vi "SCMP - System init v2.vi"(8 "error in (no error)":errorcluster, 9 "Pane Color":u32, 10 "instrument":string) -> (0 "error main":errorcluster, 1 "Cameras":refnum<class "Camera.lvclass">[](array[class]), 2 "Peripherals":T1, 3 "cont?":bool=TRUE, 5 "Today's SCMP Engineering File":path, 7 "Version":string)   [LabVIEW 2014]
uses:
  Controls/peripherals.ctl
  AISAS/Mech/AISAS Mech.lvclass
  Camera/Camera/Camera.lvclass
  Camera/Andor Neo/Andor.lvclass
  Controls/SCD - FITS Cluster.ctl
  AISAS/Controls/Diffuser.ctl
  Controls/FITS Data type.ctl
  Controls/SCD - Calibration Optics Filter Wheel.ctl
  Controls/SCD - EDT - Emission Line Filter Wheel.ctl
  Controls/CoMP-S Controls/Polarization Optics Filter Wheel.ctl
  Controls/CoMP-S Controls/Emission Line Filter Wheel.ctl
  AISAS/Controls/focus.ctl
  Controls/Cameras select.ctl
  Controls/Globals.vi
  Controls/Global demo.vi
panel:
  in  "Force PI Init":bool
  in  "Shutter":string(combo)="Global"
  in  "Temperature":string(combo)="-25.00"
  out "error eng":errorcluster
  # "System initialization\n        wait please"
  # "Peripherals"
  # "Andor control"
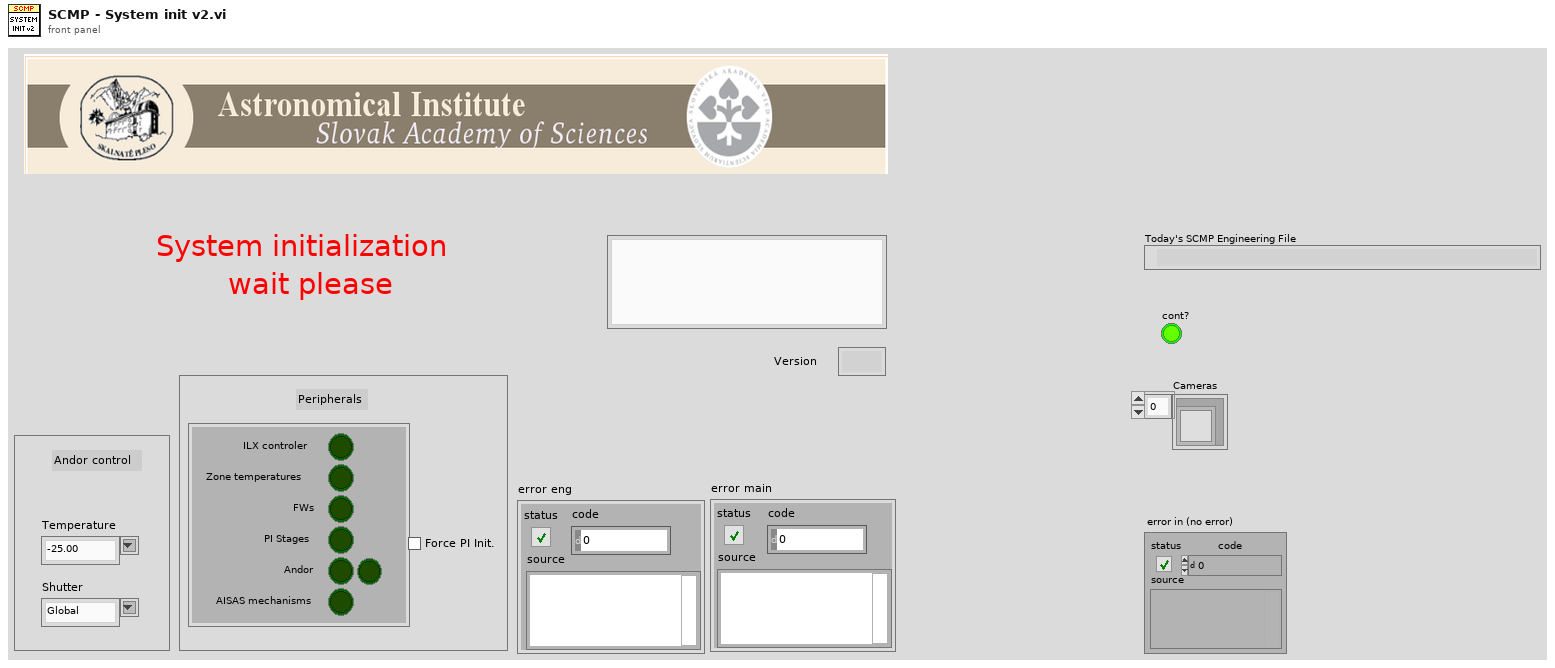
[diagram p1: front panel]
types:
  T1 = typedef "peripherals.ctl" = cluster{"ILX controler":bool, "Zone temperatures":bool, "Andor":bool, "Andor 2":bool, "PI Stages":bool, "AISAS mechanisms":bool, "AISAS Mech.lvclass":refnum<class "AISAS Mech.lvclass">, "Zone temp ref":variant, "FWs":bool}
  T2 = cluster{"server address":string, "remote port (502)":u16}
  T3 = enum32{"Invalid", "Standard", "Closed", "Hidden", "Minimized", "Maximized"}
  T4 = typedef "SCD - FITS Cluster.ctl" = cluster{"Wavelength (nm)":dbl, "Exposure (s)":dbl, "Tuning Delay (ms)":dbl, "Beam Type (-1/1)":dbl, "Tuning Voltages":dbl[], "Observer":string, "Light Shapping Diffuser":T5, "Comment":string, "Data Type":T6, "Mod Cycles":u16, "SCD Calibration Optics":T7, "SCD Emission Line Filter":T8, "Cookbook":string, "COMP-S Calibration Wheel":T9, "COMP-S Andover Filter Wheel":T10, "FOV Rotation (deg)":dbl, "Objective Lens Position (mm)":T11, "Occulter size":dbl, "Time End":timestamp, "Acc Exposure (s)":dbl, "Time Stamp Array":timestamp[], "Camera Serial Number":string[], "Camera Temp":dbl[], "Camera PI (mm)":dbl[], "Time Start":timestamp, "Peripherals":T1, "FITS paths":path[], "Cameras":T12, "load preset cbk":bool, "periodic check count":i32, "COMP-S Calibration Wheel 2":T9, "Calib":enum16{"Dark", "Flat"}, "Abso Aperture":dbl, "Nominal Aperture":dbl, "Pointer IP":string}
  T5 = typedef "Diffuser.ctl" = enum16{"Out of Beam", "In Beam"}
  T6 = typedef "FITS Data type.ctl" = enum16{"LIVE", "DARK", "FLAT", "CALI", "OBSE", "ABSO", "AURE", "TARG", "OBJE", "HOLE", "OREX", "THRO", "CHIP"}
  T7 = typedef "SCD - Calibration Optics Filter Wheel.ctl" = enum16{"1 - Polarizer @0, I+Q", "2 - Polarizer @90, I-Q", "3 - Polarizer @45, I+U", "4 - Polarizer @135, I-U", "5 - Polarizer @0, Retarder @45, I+V", "6 - Polarizer @0, Retarder @135, I-V", "7 - Dark", "8 - Clear", "9 - N/A"}
  T8 = typedef "SCD - EDT - Emission Line Filter Wheel.ctl" = enum16{"1-557.6nm", "2-587.6nm", "3-589.6nm", "4-630.2nm", "5-656.4nm", "6-849.8nm", "7-854.2nm", "8-866.2nm", "9-1083.0nm"}
  T9 = typedef "Polarization Optics Filter Wheel.ctl" = enum16{"Dark", "Clear", "Exchange Lens", "Polarizer @0, I+Q", "Polarizer @90, I-Q", "Polarizer @45, I+U", "Polarizer @135, I-U", "Polarizer @0, Retarder @45, I+V", "Polarizer @0, Retarder @135, I-V"}
  T10 = typedef "Emission Line Filter Wheel.ctl" = enum16{"530.3nm/HWB 0.34nm (Fe XIV)", "587.6nm/HBW 0.44nm (He I D3)", "637.5nm/HBW 0.53nm (Fe X)", "656.3nm/HBW 0.57nm (H-Alpha)", "789.2nm/HBW 0.85nm (Fe XI)", "854.2nm/HBW 1.01nm (Ca I)", "1074.7nm/HBW 2.34nm (Fe XIII)", "1079.8nm/HBW 1.64nm (Fe XIII)", "1083.0nm/HBW 1.66nm (He I)"}
  T11 = typedef "focus.ctl" = dbl
  T12 = typedef "Cameras select.ctl" = enum16{"Andor", "GDR"}
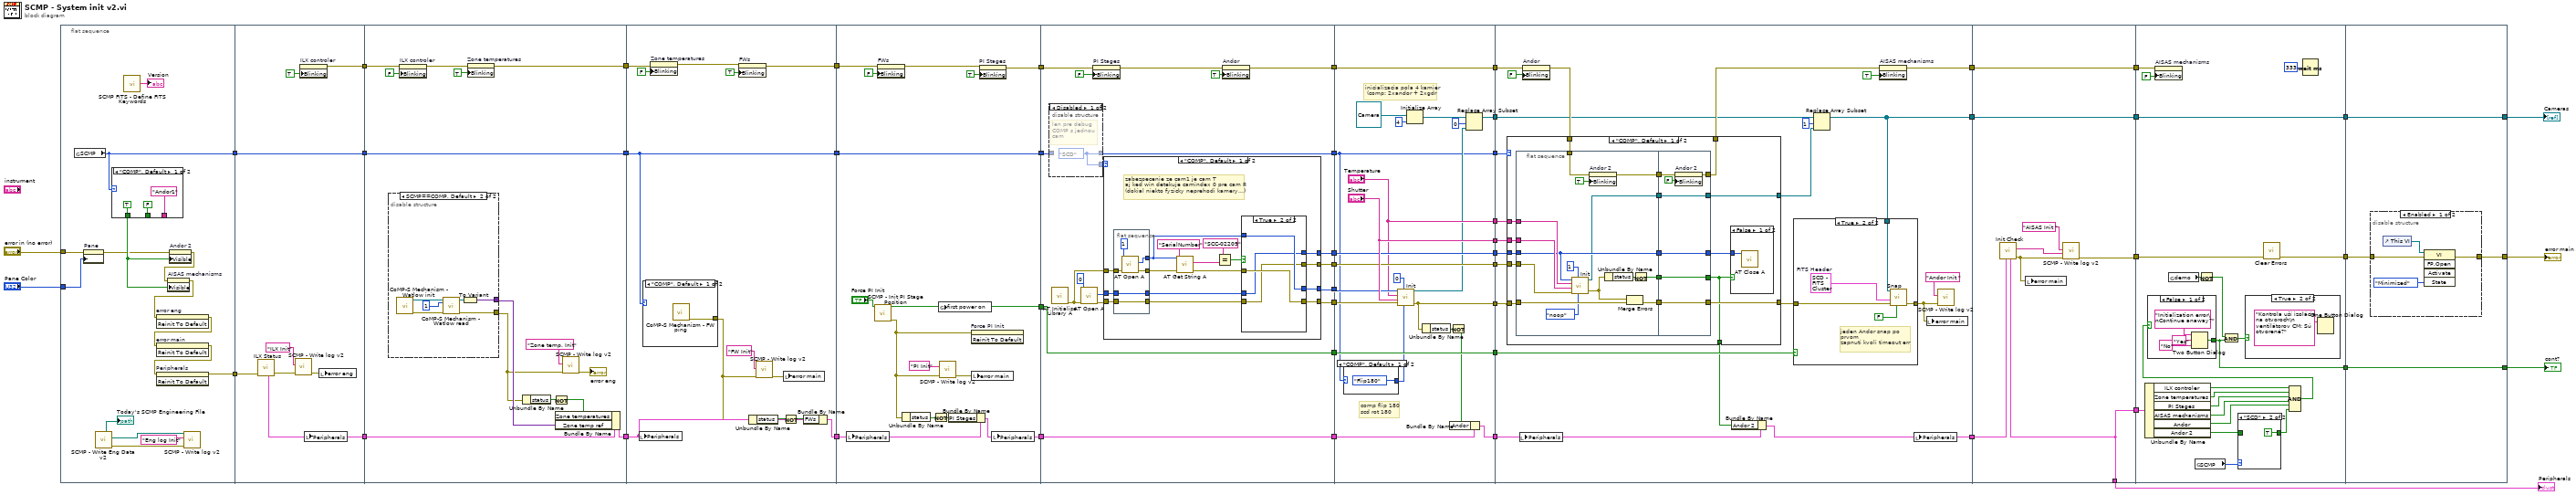
[diagram p0: block diagram]
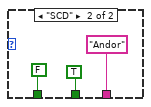
[diagram p2: hidden frame]
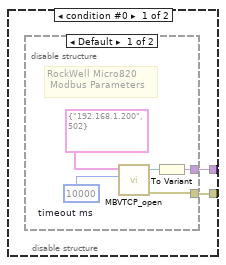
[diagram p3: hidden frame]
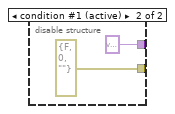
[diagram p4: hidden frame]
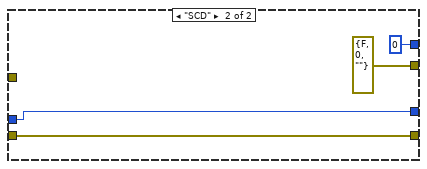
[diagram p8: hidden frame]
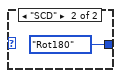
[diagram p9: hidden frame]
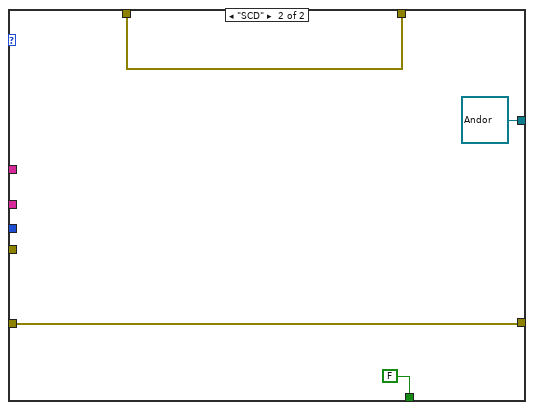
[diagram p11: hidden frame]
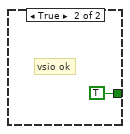
[diagram p15: hidden frame]
diagram:
  n1 = flat-sequence {
    tunnel: [w62] -> w41
    tunnel: [w50] -> w24
    tunnel: "error in (no error)" -> [w58]
    tunnel: "Pane Color" -> [w57]
    tunnel: [w71] -> w14
    tunnel: [w77] -> w13
    tunnel: w41 -> [w76]
    tunnel: w24 -> [w75]
    tunnel: [w75] -> w12
    tunnel: w14 -> [w90]
    tunnel: [w89] -> w44
    tunnel: [w87] -> w42
    tunnel: [w85] -> w21
    tunnel: w12 -> [w85]
    tunnel: w13 -> [w83]
    tunnel: w44 -> [w113]
    tunnel: [w114] -> w43
    tunnel: w42 -> [w118]
    tunnel: [w112] -> w22
    tunnel: w21 -> [w112]
    tunnel: [w115] -> w11
    tunnel: w43 -> [w128]
    tunnel: [w134] -> w32
    tunnel: [w129] -> w23
    tunnel: w22 -> [w129]
    tunnel: w11 -> [w125]
    tunnel: [w123] -> w10
    tunnel: [w121] -> w9
    tunnel: [w142] -> w40
    tunnel: [w150] -> w39
    tunnel: [w147] -> w36
    tunnel: [w146] -> w35
    tunnel: [w145] -> w34
    tunnel: [w144] -> w33
    tunnel: w32 -> [w136]
    tunnel: [w136] -> w31
    tunnel: w23 -> [w138]
    tunnel: w10 -> [w140]
    tunnel: w9 -> [w142]
    tunnel: [w137] -> w8
    tunnel: [w199] -> w49
    tunnel: [w211] -> w48
    tunnel: ["Shutter"] -> w47
    tunnel: ["Temperature"] -> w46
    tunnel: w40 -> [w209]
    tunnel: [w208] -> w45
    tunnel: w39 -> [w208]
    tunnel: [w204] -> w38
    tunnel: [w205] -> w37
    tunnel: w36 -> [w207]
    tunnel: w35 -> [w206]
    tunnel: w34 -> [w205]
    tunnel: w33 -> [w204]
    tunnel: w31 -> [w203]
    tunnel: [w203] -> w30
    tunnel: [w191] -> w20
    tunnel: w8 -> [w191]
    tunnel: [w192] -> w6
    tunnel: w49 -> [w236]
    tunnel: [w225] -> w27
    tunnel: w48 -> [w232]
    tunnel: w47 -> [w234]
    tunnel: w46 -> [w233]
    tunnel: w45 -> [w231]
    tunnel: w38 -> [w229]
    tunnel: w37 -> [w228]
    tunnel: w30 -> [w227]
    tunnel: [w220] -> w25
    tunnel: w20 -> [w219]
    tunnel: w6 -> [w217]
    tunnel: [w214] -> w4
    tunnel: [w293] -> w28
    tunnel: w27 -> [w288]
    tunnel: [w292] -> w26
    tunnel: w25 -> [w292]
    tunnel: [w286] -> w19
    tunnel: [w287] -> w5
    tunnel: w4 -> [w287]
    tunnel: [w286] -> w1
    tunnel: w28 -> [w299]
    tunnel: w26 -> [w311]
    tunnel: w19 -> [w300]
    tunnel: [w298] -> w16
    tunnel: [w303] -> w15
    tunnel: w5 -> [w297]
    tunnel: [w297] -> w3
    tunnel: [w325] -> w29
    tunnel: w16 -> [w324]
    tunnel: w15 -> [w325]
    tunnel: [w323] -> w7
    tunnel: [w322] -> w2
    tunnel: w3 -> [w322]
    frame #0 {
      n2 = global read "Globals.vi" "SCMP"() -> (w50:enum16{"COMP", "SCD"})
      n3 = property on="Pane" class="Pane"(error in=w58, "PaneColor"=w57) -> (error out=w51:errorcluster)  [unwired: 1 in, 1 out]
      n4 = call "SCMP - Write Eng Data v2.vi"() -> ("error out"=w52:errorcluster, "Today's SCMP folder"=w55:path, "Today's SCMP Engineering File"=→"Today's SCMP Engineering File":path)  [unwired: 8 in, 1 out]
      n5 = case shown="\"COMP\", Default" w50 {
        tunnel: ["Andor1" ("Caption.Text") "Andor" ("Caption.Text")] -> _
        tunnel: [FALSE ("Caption.Visible") TRUE ("Caption.Visible")] -> _
        tunnel: [TRUE ("Caption.Visible") FALSE ("Caption.Visible")] -> w60
        frame "COMP", Default {
        }
        frame "SCD" {
        }
      }
      n6 = call "SCMP FITS - Define FITS Keywords.vi"() -> ("Version"=→"Version":string)  [unwired: 5 in, 6 out]
      n7 = property on="Andor 2" class="Bool (strict)"(error in=w51, "Visible"=w60) -> (error out=w61:errorcluster)  [unwired: 1 in, 1 out]
      n8 = property on="AISAS mechanisms" class="Bool (strict)"(error in=w61, "Visible"=w60) -> (error out=w59:errorcluster)  [unwired: 1 in, 1 out]
      n9 = invoke on="error eng" class="Clust (strict)" method="Reinit To Default"(error in=w59) -> (error out=w64:errorcluster)  [unwired: 2 in, 2 out]
      n10 = invoke on="error main" class="Clust (strict)" method="Reinit To Default"(error in=w64) -> (error out=w63:errorcluster)  [unwired: 2 in, 2 out]
      n11 = invoke on="Peripherals" class="Clust (strict)" method="Reinit To Default"(error in=w63) -> (error out=w62:errorcluster)  [unwired: 2 in, 2 out]
      n12 = call "SCMP - Write log v2.vi"("Error to log"=w52, "data"="Eng log Init" ("mesage"), "Today's SCMP folder"=w55) -> ()  [unwired: 6 in, 3 out]
    }
    frame #1 {
      n13 = call "ILX Status.vi"("error in"=w76) -> ("error out"=w74:errorcluster, "Peripherals out"=w71:T1)  [unwired: 5 in, 4 out]
      n14 = call "SCMP - Write log v2.vi"("Error to log"=w74, "data"="ILX Init" ("mesage")) -> ("error out"=w72:errorcluster)  [unwired: 7 in, 2 out]
      n15 = property on="ILX controler" class="Bool (strict)"("Blinking"=TRUE) -> (error out=w77:errorcluster)  [unwired: 2 in, 1 out]
      n16 = local write "Peripherals"(w71) -> ()
      n17 = local write "error eng"(w72) -> ()
    }
    frame #2 {
      n18 = disable-structure shown="SCMP==COMP, Default" {
        disable-tunnel: [w94 w102] -> w80
        disable-tunnel: [w93 w103] -> w86
        frame condition #0 {
          n19 = disable-structure shown="Default" {
            disable-tunnel: [w95 errorcluster {"status"=FALSE, "code"=0, "source"=""} ("error in")] -> w94
            disable-tunnel: [w96 variant ("Variant")] -> w93
            frame condition #0 {
              w98 = 10000  # timeout ms
              # "RockWell Micro820\n Modbus Parameters"
              n20 = call <vilib>:"MBVTCP_open.vi"("timeout ms (60000)"=w98, "Network"=T2 {"server address"="192.168.1.200", "remote port (502)"=502} ("Rockwell Address and Port")) -> ("error out"=w95:errorcluster, "NetRefTCP out"=w97:refnum<k5>)  [unwired: 1 in, 7 out]
              n21 = To Variant(anything=w97) -> (Variant=w96:variant)
            }
            frame condition #1 (active) {
            }
          }
        }
        frame condition #1 (active) {
          n22 = call "CoMP-S Mechanism - Watlow init.vi"() -> ("error out"=w104:errorcluster, "ILabVIEW"=w105:refnum<k24>)  [unwired: 8 in, 1 out]
          n23 = call "CoMP-S Mechanism - Watlow read.vi"("6. Instance ID"=1, "error in (no error)"=w104, "ILabVIEW In"=w105) -> ("error out"=w102:errorcluster)  [unwired: 4 in, 2 out]
          n24 = To Variant(anything=w105) -> (Variant=w103:variant)
        }
      }
      n25 = property on="ILX controler" class="Bool (strict)"(error in=w83, "Blinking"=FALSE) -> (error out=w82:errorcluster)  [unwired: 1 in, 1 out]
      n26 = property on="Zone temperatures" class="Bool (strict)"(error in=w82, "Blinking"=TRUE) -> (error out=w87:errorcluster)  [unwired: 1 in, 1 out]
      n27 = Unbundle By Name(w80) -> ("status"=w92:bool)
      n28 = Not(x=w92) -> (.not. x?=w88:bool)
      n29 = Bundle By Name(cluster=w90, "Zone temperatures"=w88, "Zone temp ref"=w86) -> (w89:T1)
      n30 = call "SCMP - Write log v2.vi"("Error to log"=w80, "data"="Zone temp. Init" ("mesage")) -> ("error out"=→"error eng":errorcluster)  [unwired: 7 in, 2 out]
    }
    frame #3 {
      n31 = local write "Peripherals"(w113) -> ()
      n32 = case shown="\"COMP\", Default" w112 {
        tunnel: [w120 _] -> w109
        frame "COMP", Default {
          n33 = call "CoMP-S Mechanism - FW ping.vi"() -> ("error out"=w120:errorcluster)  [unwired: 10 in, 1 out]
        }
        frame "SCD" {
        }
      }
      n34 = property on="Zone temperatures" class="Bool (strict)"(error in=w118, "Blinking"=FALSE) -> (error out=w116:errorcluster)  [unwired: 1 in, 1 out]
      n35 = property on="FWs" class="Bool (strict)"(error in=w116, "Blinking"=TRUE) -> (error out=w115:errorcluster)  [unwired: 1 in, 1 out]
      n36 = Unbundle By Name(w109) -> ("status"=w111:bool)
      n37 = call "SCMP - Write log v2.vi"("Error to log"=w109, "data"="FW Init" ("mesage")) -> ("error out"=w107:errorcluster)  [unwired: 7 in, 2 out]
      n38 = Not(x=w111) -> (.not. x?=w110:bool)
      n39 = local write "error main"(w107) -> ()
      n40 = Bundle By Name(cluster=w113, "FWs"=w110) -> (w114:T1)
    }
    frame #4 {
      n41 = local write "Peripherals"(w128) -> ()
      n42 = call "SCMP - Init PI Stage Position.vi"("Force PI Init"="Force PI Init") -> ("error out"=w122:errorcluster, "first power on"=w134:bool)  [unwired: 9 in]
      n43 = property on="FWs" class="Bool (strict)"(error in=w125, "Blinking"=FALSE) -> (error out=w124:errorcluster)  [unwired: 1 in, 1 out]
      n44 = Unbundle By Name(w122) -> ("status"=w133:bool)
      n45 = Not(x=w133) -> (.not. x?=w132:bool)
      n46 = global write "Globals.vi" "first power on"(w134) -> ()
      n47 = call "SCMP - Write log v2.vi"("Error to log"=w122, "data"="PI Init" ("mesage")) -> ("error out"=w130:errorcluster)  [unwired: 7 in, 2 out]
      n48 = Bundle By Name(cluster=w128, "PI Stages"=w132) -> (w121:T1)
      n49 = invoke on="Force PI Init" class="Bool (strict)" method="Reinit To Default"(error in=w122) -> ()  [unwired: 2 in, 3 out]
      n50 = local write "error main"(w130) -> ()
      n51 = property on="PI Stages" class="Bool (strict)"(error in=w124, "Blinking"=TRUE) -> (error out=w123:errorcluster)  [unwired: 1 in, 1 out]
      n52 = local write "Peripherals"(w121) -> ()
    }
    frame #5 {
      n53 = disable-structure shown="Disabled" {
        disable-tunnel: [w154 w155] -> w139
        disable-tunnel: w138 -> [_ w155]
        disable-tunnel: [w154 w155] -> w137
        frame Disabled {
          w154 = enum16{"COMP", "SCD"}."SCD" ("SCMP")
          # "len pre debug\nCOMP s jednou\ncam"
        }
        frame Enabled {
        }
      }
      n54 = call <userlib>:"AT Initialise Library A.vi"() -> ("error out"=w141:errorcluster)  [unwired: 10 in, 1 out]
      n55 = call <userlib>:"AT Open A.vi"("error in (no error)"=w141, "CameraIndex"=0) -> ("error out"=w148:errorcluster, "Handle"=w143:i32)  [unwired: 7 in, 1 out]
      n56 = property on="PI Stages" class="Bool (strict)"(error in=w140, "Blinking"=FALSE) -> (error out=w153:errorcluster)  [unwired: 1 in, 1 out]
      n57 = case shown="\"COMP\", Default" w139 {
        tunnel: w148 -> [w171 w188]
        tunnel: [w170 w189] -> w147
        tunnel: [w169 w188] -> w146
        tunnel: [w168 0 ("Handle")] -> w145
        tunnel: [w167 errorcluster {"status"=FALSE, "code"=0, "source"=""} ("error out")] -> w144
        tunnel: w143 -> [w166 w189]
        tunnel: w141 -> [w165 _]
        frame "COMP", Default {
          # "zabezpecenie ze cam1 je cam T\naj ked win detekuje camindex 0 pre cam R\n(dokial niekto fyzicky neprehodi kamery...)"
          n58 = flat-sequence {
            tunnel: w171 -> [w183]
            tunnel: [w184] -> w163
            tunnel: [w181] -> w156
            tunnel: w166 -> [w182]
            tunnel: [w183] -> w158
            tunnel: [w182] -> w157
            tunnel: w165 -> [w180]
            frame #0 {
              n59 = call <userlib>:"AT Open A.vi"("error in (no error)"=w180, "CameraIndex"=1) -> ("error out"=w184:errorcluster, "Handle"=w181:i32)  [unwired: 7 in, 1 out]
            }
          }
          n60 = call <userlib>:"AT Get String A.vi"("error in (no error)"=w163, "Feature"="SerialNumber", "Handle"=w156) -> ("error out"=w159:errorcluster, "String"=w162:string)  [unwired: 6 in, 1 out]
          n61 = Equal?(x="SCC-02209", y=w162) -> (x = y?=w160:bool)
          n62 = case shown="True" w160 {
            tunnel: w159 -> [w173 w178]
            tunnel: w158 -> [w175 w176]
            tunnel: w157 -> [w174 w177]
            tunnel: w156 -> [w172 w179]
            tunnel: [w174 w179] -> w170
            tunnel: [w175 w178] -> w169
            tunnel: [w172 w177] -> w168
            tunnel: [w173 w176] -> w167
            frame False {
            }
            frame True {
            }
          }
        }
        frame "SCD" {
        }
      }
      n63 = property on="Andor" class="Bool (strict)"(error in=w153, "Blinking"=TRUE) -> (error out=w150:errorcluster)  [unwired: 1 in, 1 out]
    }
    frame #6 {
      # "comp flip 180\nscd rot 180"
      # "inicializacia pola 4 kamier\n (comp: 2xandor + 2xgdr"
      n64 = case shown="\"COMP\", Default" w191 {
        tunnel: [enum16{"noop", "Rot180", "Flip180"}."Flip180" ("op (noop)") enum16{"noop", "Rot180", "Flip180"}."Rot180" ("op (noop)")] -> w190
        frame "COMP", Default {
        }
        frame "SCD" {
        }
      }
      n65 = call "Init.vi"("rot/flip"=w190, "Camera Index"=0 ("CameraIndex"), "error in"=w206, "Shutter"="Shutter", "Temperature"="Temperature", "Neo Handle"=w207) -> ("error out"=w199:errorcluster, "Andor.lvclass"=w195:refnum<class "Andor.lvclass">)  [unwired: 4 in]
      n66 = Initialize Array(refnum<class "Camera.lvclass"> refnum ("Camera.lvclass"), 4 ("dimension size")) -> (w196:refnum<class "Camera.lvclass">[])
      n67 = Unbundle By Name(w199) -> ("status"=w200:bool)
      n68 = Not(x=w200) -> (.not. x?=w198:bool)
      n69 = Bundle By Name(cluster=w209, "Andor"=w198) -> (w211:T1)
      n70 = Replace Array Subset(array=w196, new element=w195, index=0) -> (w192:refnum<class "Camera.lvclass">[])
    }
    frame #7 {
      n71 = local write "Peripherals"(w232) -> ()
      n72 = property on="Andor" class="Bool (strict)"(error in=w231, "Blinking"=FALSE) -> (error out=w223:errorcluster)  [unwired: 1 in, 1 out]
      n73 = case shown="\"COMP\", Default" w219 {
        tunnel: w236 -> [w248 w278]
        tunnel: w234 -> [w247 _]
        tunnel: w233 -> [w246 _]
        tunnel: [w245 w278] -> w230
        tunnel: w229 -> [w244 _]
        tunnel: w228 -> [w243 _]
        tunnel: w223 -> [w242 w279]
        tunnel: [w241 w279] -> w221
        tunnel: [w238 FALSE] -> w218
        tunnel: [w237 refnum<class "Andor.lvclass"> refnum ("Andor.lvclass")] -> w215
        frame "COMP", Default {
          n74 = flat-sequence {
            tunnel: [w267] -> w252
            tunnel: w248 -> [w268]
            tunnel: [w258] -> w251
            tunnel: w247 -> [w265]
            tunnel: w246 -> [w263]
            tunnel: w244 -> [w264]
            tunnel: w243 -> [w260]
            tunnel: w242 -> [w262]
            tunnel: [w261] -> w250
            tunnel: [w260] -> w249
            tunnel: [w255] -> w239
            tunnel: [w273] -> w245
            tunnel: w252 -> [w273]
            tunnel: [w275] -> w237
            tunnel: w251 -> [w275]
            tunnel: w250 -> [w272]
            tunnel: [w271] -> w241
            tunnel: w249 -> [w270]
            tunnel: [w270] -> w240
            tunnel: [w269] -> w238
            tunnel: w239 -> [w269]
            frame #0 {
              n75 = call "Init.vi"("rot/flip"=enum16{"noop", "Rot180", "Flip180"}."noop" ("Rotation"), "Camera Index"=1 ("CameraIndex"), "error in"=w264, "Shutter"=w265, "Temperature"=w263, "Neo Handle"=w260) -> ("error out"=w256:errorcluster, "Andor.lvclass"=w258:refnum<class "Andor.lvclass">)  [unwired: 4 in]
              n76 = property on="Andor 2" class="Bool (strict)"(error in=w262, "Blinking"=TRUE) -> (error out=w261:errorcluster)  [unwired: 1 in, 1 out]
              n77 = Unbundle By Name(w256) -> ("status"=w257:bool)
              n78 = Merge Errors(w256, w268) -> (w267:errorcluster)
              n79 = Not(x=w257) -> (.not. x?=w255:bool)
            }
            frame #1 {
              n80 = property on="Andor 2" class="Bool (strict)"(error in=w272, "Blinking"=FALSE) -> (error out=w271:errorcluster)  [unwired: 1 in, 1 out]
            }
          }
          n81 = case shown="False" w238 {
            tunnel: w240 -> [w253 _]
            frame False {
              n82 = call <userlib>:"AT Close A.vi"("Handle"=w253) -> ()  [unwired: 9 in, 2 out]
            }
            frame True {
            }
          }
        }
        frame "SCD" {
        }
      }
      n83 = Bundle By Name(cluster=w232, "Andor 2"=w218) -> (w225:T1)
      n84 = Replace Array Subset(array=w217, new element=w215, index=1) -> (w214:refnum<class "Camera.lvclass">[])
      n85 = case shown="True" w227 {
        tunnel: w230 -> [w280 w285]
        tunnel: [w280 w284] -> w226
        tunnel: w214 -> [_ w281]
        frame False {
        }
        frame True {
          w283 = T4 {"Wavelength (nm)"=0.0, "Exposure (s)"=0.0, "Tuning Delay (ms)"=0.0, "Beam Type (-1/1)"=0.0, "Tuning Voltages"=[], "Observer"="", "Light Shapping Diffuser"=enum."Out of Beam", "Comment"="", "Data Type"=enum."LIVE", "Mod Cycles"=0, "SCD Calibration Optics"=enum."1 - Polarizer @0, I+Q", "SCD Emission Line Filter"=enum."1-557.6nm", "Cookbook"="", "COMP-S Calibration Wheel"=enum."Dark", "COMP-S Andover Filter Wheel"=enum."530.3nm/HWB 0.34nm (Fe XIV)", "FOV Rotation (deg)"=0.0, "Objective Lens Position (mm)"=0.0, "Occulter size"=0.0, "Time End"=timestamp(0 s since 1904-01-01), "Acc Exposure (s)"=0.0, "Time Stamp Array"=[], "Camera Serial Number"=[], "Camera Temp"=[], "Camera PI (mm)"=[], "Time Start"=timestamp(3382374145.421875 s since 1904-01-01), "Peripherals"={"ILX controler"=FALSE, "Zone temperatures"=FALSE, "Andor"=FALSE, "Andor 2"=FALSE, "PI Stages"=FALSE, "AISAS mechanisms"=FALSE, "AISAS Mech.lvclass"=refnum, "Zone temp ref"=variant, "FWs"=FALSE}, "FITS paths"=[], "Cameras"=enum."Andor", "load preset cbk"=FALSE, "periodic check count"=0, "COMP-S Calibration Wheel 2"=enum."Dark", "Calib"=enum."Dark", "Abso Aperture"=66.0, "Nominal Aperture"=66.0, "Pointer IP"="127.0.0.1"}  # FITS Header
          # "jeden Andor snap po prvom \nzapnuti kvoli timeout err"
          n86 = call "Snap.vi"("Save Data to FITS? (F)"=FALSE, "error in"=w285, "FITS/UI"=w283, "Cameras in"=w281) -> ("error out"=w284:errorcluster)  [unwired: 4 in, 3 out]
        }
      }
      n87 = property on="AISAS mechanisms" class="Bool (strict)"(error in=w221, "Blinking"=TRUE) -> (error out=w220:errorcluster)  [unwired: 1 in, 1 out]
      n88 = local write "Peripherals"(w225) -> ()
      n89 = local write "error main"(w226) -> ()
      n90 = call "SCMP - Write log v2.vi"("Error to log"=w226, "data"="Andor Init ") -> ()  [unwired: 7 in, 3 out]
    }
    frame #8 {
      n91 = call "Init Check.vi"("Peripherals in"=w288) -> ("error out"=w291:errorcluster, "auto off resp"=w289:string, "Peripherals out"=w286:T1)  [unwired: 7 in, 1 out]
      n92 = local write "error main"(w291) -> ()
      n93 = call "SCMP - Write log v2.vi"("Error to log"=w291, "data to end"=w289, "data"="AISAS Init ") -> ("error out"=w293:errorcluster)  [unwired: 6 in, 2 out]
    }
    frame #9 {
      n94 = Unbundle By Name(w300) -> ("ILX controler"=w310:bool, "Zone temperatures"=w309:bool, "PI Stages"=w308:bool, "AISAS mechanisms"=w307:bool, "Andor"=w306:bool, "Andor 2"=w295:bool)
      n95 = property on="AISAS mechanisms" class="Bool (strict)"(error in=w311, "Blinking"=FALSE) -> ()  [unwired: 1 in, 2 out]
      n96 = global read "Global demo.vi" "demo"() -> (w304:bool)
      n97 = global read "Globals.vi" "SCMP"() -> (w296:enum16{"COMP", "SCD"})
      n98 = Not(x=w304) -> (.not. x?=w301:bool)
      n99 = case shown="\"SCD\"" w296 {
        tunnel: w295 -> [w314 _]
        tunnel: [w314 TRUE ("Andor 2")] -> w294
        frame "COMP", Default {
        }
        frame "SCD" {
        }
      }
      n100 = call <vilib>:"Clear Errors.vi"("error in (no error)"=w299) -> ("error out"=w298:errorcluster)  [unwired: 5 in, 1 out]
      n101 = Compound Arithmetic op=AND(w310, w309, w308, w307, w306, w294) -> (w305:bool)
      n102 = case shown="False" w305 {
        tunnel: [w317 TRUE ("T button?")] -> w303
        frame False {
          n103 = Two Button Dialog(message="Initialization error\nContinue anaway?", 1:"No" ("F button name (\"Cancel\")"), 2:"Yes" ("T button name (\"OK\")")) -> (T button?=w317:bool)
        }
        frame True {
          # "vsio ok"
        }
      }
      n104 = And(x=w301, y=w303) -> (x .and. y?=w302:bool)
      n105 = case shown="True" w302 {
        frame False {
        }
        frame True {
          n106 = One Button Dialog(message="Kontrola uší izolácie na otvoroch\n  ventilátorov CM: Sú otvorené?") -> ()  [unwired: 1 in, 1 out]
        }
      }
      n107 = Wait (ms)(milliseconds to wait=u32 333) -> ()  [unwired: 1 out]
    }
    frame #10 {
      n108 = disable-structure shown="Enabled" {
        disable-tunnel: w324 -> [w327 _]
        disable-tunnel: [w326 _] -> w323
        frame Enabled {
          n109 = control-ref of="This VI"() -> (w328:refnum<vi>)
          n110 = invoke class="VI" method="FP.Open"(reference=w328, error in=w327, "State"=T3."Minimized") -> (error out=w326:errorcluster)  [unwired: 2 in, 4 out]
        }
        frame Disabled {
        }
      }
    }
  }
  "error main" <- w7
  "cont?" <- w29
  "Cameras" <- w2
  "Peripherals" <- w1
